vi "final16.vi"() -> ()   [LabVIEW 2019]
uses:
  <vilib>/Instr/_visa.llb/VISA Configure Serial Port (Instr).vi
  <vilib>/Analysis/NI_AALPro.lvlib
  <vilib>/Analysis/NI_AALBase.lvlib
panel:
  out "residue_gain0":dbl
  out "residue_gain2":dbl
  out "residue_gain1":dbl
  out "Received data":string
  out "initialized array":dbl[](array[numeric])
  out "standard deviation":dbl format="%0.2f"
  out "variance":dbl format="%0.2f"
  out "mean":dbl format="%0.2f"
  out "Conversion [g]":dbl
  out "slope_gain0":dbl
  out "intercept_gain0":dbl
  out "slope_gain2":dbl
  out "intercept_gain2":dbl
  out "slope_gain1":dbl
  out "intercept_gain1":dbl
  out "Debug array":string[](array[string])
  in  "Stop":bool
  in  "Cycles":dbl min=1.0 step=1.0
  in  "Start operation":bool
  out "String passed to Arduino":string
  in  "Function":u16(ring) items=["Read data ", "Compare different gains", "Execute calibration"]
  in  "Gain":u16(ring) items=["32", "64", "128"]
  in  "Arduino COM port":refnum<visa-resource-name>="COM6"
  # "Select all options, then press \"Start operation\" button"
  # "Nerd zone"
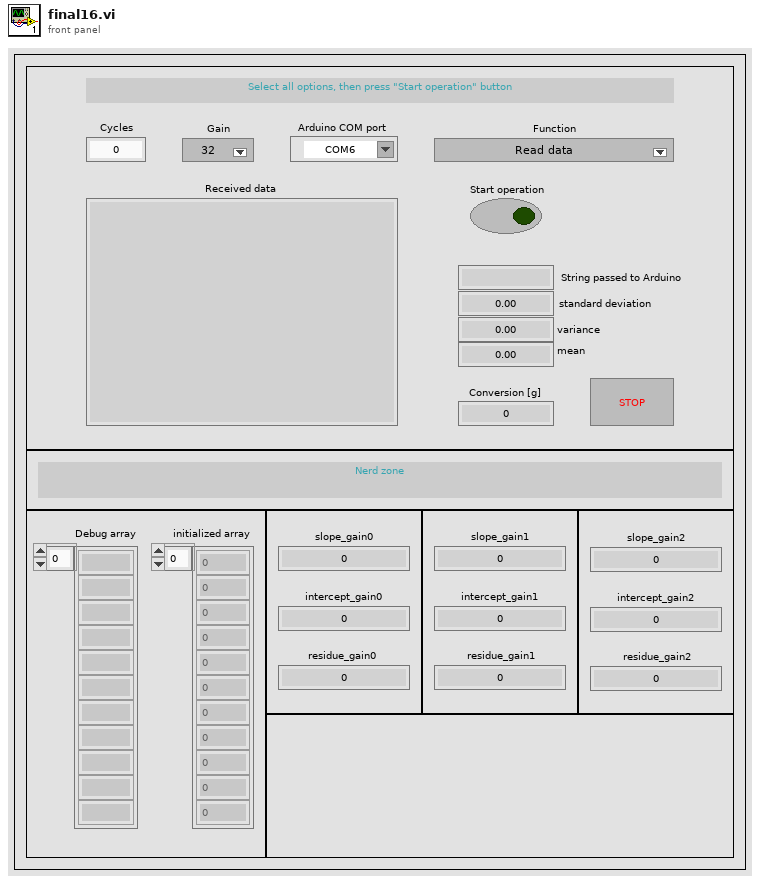
[diagram p1: front panel]
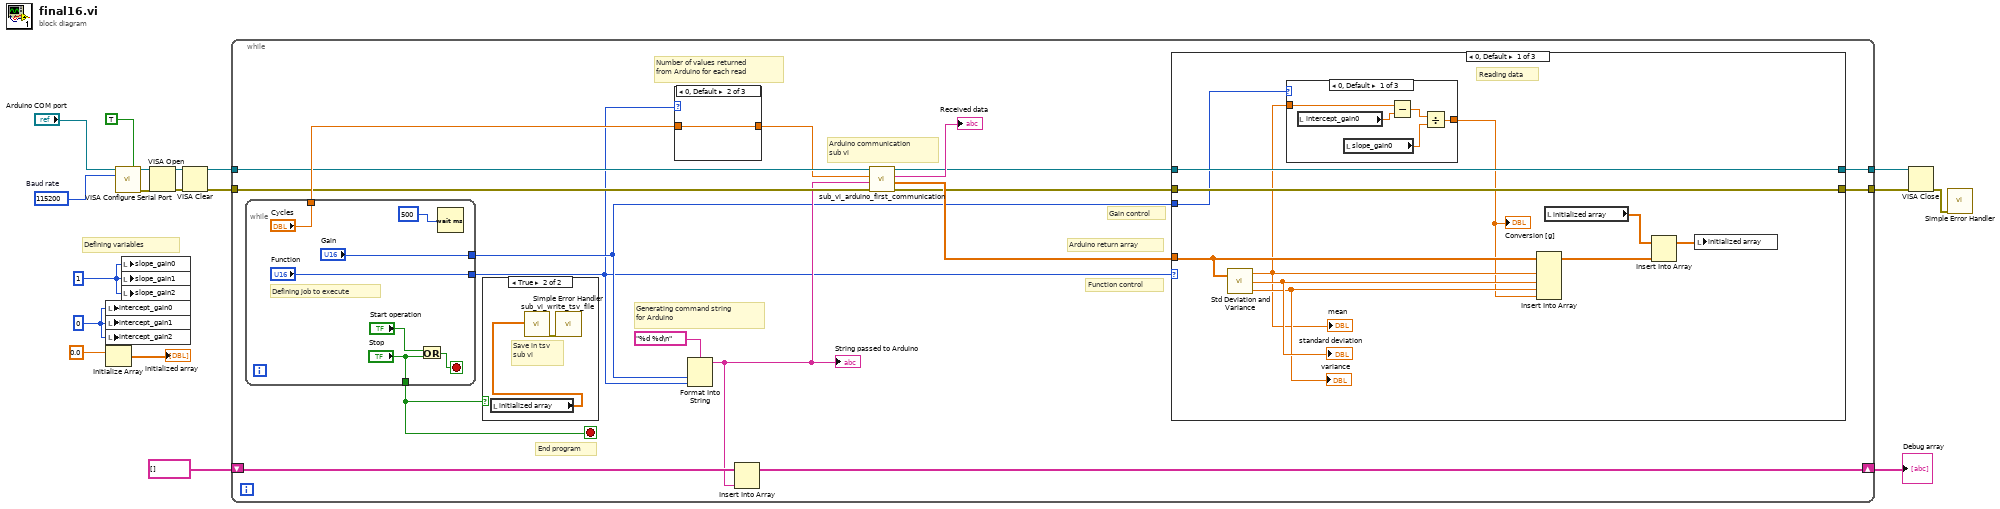
[diagram p0: block diagram]
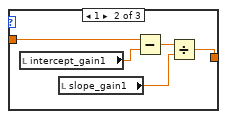
[diagram p2: hidden frame]
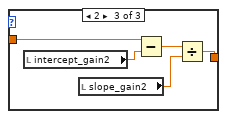
[diagram p3: hidden frame]
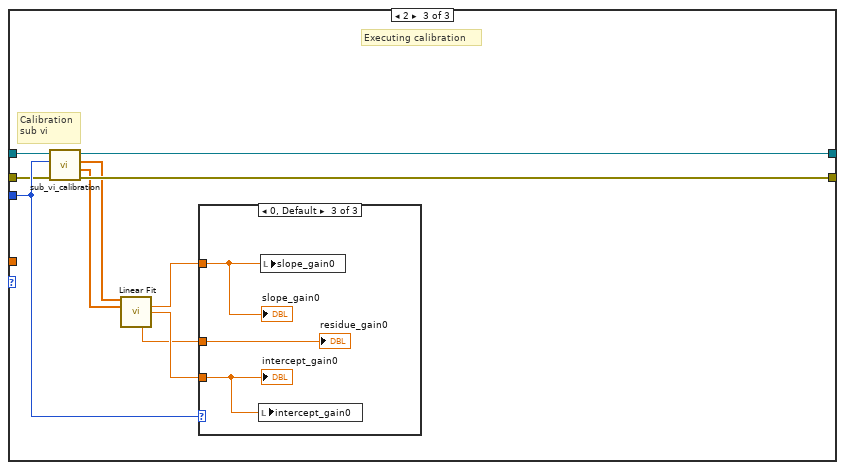
[diagram p5: hidden frame]
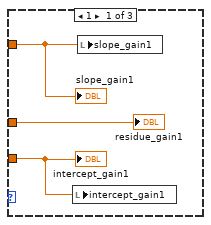
[diagram p6: hidden frame]
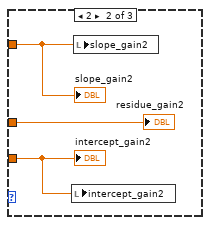
[diagram p7: hidden frame]
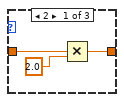
[diagram p8: hidden frame]
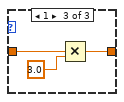
[diagram p9: hidden frame]
diagram:
  w6 = 0
  w5 = 1
  w17 = u32 115200  # Baud rate
  # "Defining variables"
  n1 = local write "intercept_gain0"(w6) -> ()
  n2 = local write "intercept_gain1"(w6) -> ()
  n3 = local write "intercept_gain2"(w6) -> ()
  n4 = Initialize Array(0.0) -> (→"initialized array":dbl[])  [unwired: 1 in]
  n5 = call-poly "VISA Configure Serial Port"("VISA resource name"="Arduino COM port", "Enable Termination\nChar (T)"=TRUE ("Enable Termination\nChar (T)"), "baud rate (9600)"=w17) -> ("VISA resource name out"=w15:refnum<visa-resource-name>, "error out"=w16:errorcluster)  [unwired: 11 in]
  n6 = local write "slope_gain0"(w5) -> ()
  n7 = local write "slope_gain1"(w5) -> ()
  n8 = local write "slope_gain2"(w5) -> ()
  n9 = VISA Open(error in (no error)=w16, VISA resource name=w15) -> (VISA resource name=w12:refnum<visa-resource-name>, error out=w13:errorcluster)  [unwired: 3 in]
  n10 = VISA Clear(VISA resource name=w12, error in (no error)=w13) -> (VISA resource name out=w10:refnum<visa-resource-name>, error out=w11:errorcluster)
  n11 = while {
    tunnel: w11 -> [w29]
    tunnel: w10 -> [w30]
    shift-right: [w35] -> w8
    shift-left: string[] [] -> [w33]
    tunnel: [w21] -> w2
    tunnel: [w22] -> w1
    stop <- w34 stop-if-true
    # "Number of values returned \nfrom Arduino for each read"
    # "End program"
    # "Generating command string\nfor Arduino"
    # "Function control"
    # "Arduino return array"
    # "Gain control"
    # "Arduino communication\nsub vi"
    n12 = while {
      tunnel: ["Function"] -> w19
      tunnel: ["Gain"] -> w20
      tunnel: ["Cycles"] -> w32
      tunnel: ["Stop"] -> w34
      stop <- w93 stop-if-true
      # "Defining job to execute"
      n13 = Or(x="Start operation", y="Stop") -> (x .or. y?=w93:bool)
      n14 = Wait (ms)(milliseconds to wait=u32 500) -> ()  [unwired: 1 out]
    }
    n15 = case shown="True" w34 {
      frame False {
      }
      frame True {
        # "Save in tsv\nsub vi"
        n16 = local read "initialized array"() -> (w90:dbl[])
        n17 = call "sub_vi_write_tsv_file.vi"("1D data"=w90) -> ("error out"=w91:errorcluster)  [unwired: 10 in]
        n18 = call <vilib>:"Simple Error Handler.vi"("error in (no error)"=w91) -> ()  [unwired: 4 in, 5 out]
      }
    }
    n19 = case shown="0, Default" w19 {
      tunnel: w32 -> [w85 w86 w87]
      tunnel: [w83 w86 w88] -> w27
      frame 2 {
        n20 = Multiply(x=w85, y=2.0) -> (x*y=w83:dbl)
      }
      frame 0, Default {
      }
      frame 1 {
        n21 = Multiply(x=w87, y=3.0) -> (x*y=w88:dbl)
      }
    }
    n22 = Format Into String(format string="%d %d\n", w20, w19) -> (resulting string=w28:string)  [unwired: 2 in, 1 out]
    "String passed to Arduino" <- w28
    n23 = Insert Into Array(array=w33, new element=w28) -> (w35:string[])  [unwired: 1 in]
    n24 = call "sub_vi_arduino_first_communication.vi"("error in (no error)"=w29, "write buffer"=w28, "Reads number"=w27, "VISA resource name in"=w30) -> ("error out"=w23:errorcluster, "Reads array"=w25:dbl[], "Received data"=→"Received data":string, "VISA resource name out"=w24:refnum<visa-resource-name>)  [unwired: 4 in]
    n25 = case shown="0, Default" w19 {
      tunnel: w20 -> [w37 _ w69]
      tunnel: w25 -> [w46 _ _]
      tunnel: w24 -> [w40 w63 w70]
      tunnel: w23 -> [w39 w62 w68]
      tunnel: [w40 w63 w64] -> w22
      tunnel: [w39 w62 w67] -> w21
      frame 0, Default {
        # "Reading data"
        n26 = call <vilib>:"Std Deviation and Variance.vi"("X"=w46) -> ("mean"=w38:dbl, "standard deviation"=w45:dbl, "variance"=w44:dbl)  [unwired: 1 in]
        "standard deviation" <- w45
        "variance" <- w44
        "mean" <- w38
        n27 = case shown="0, Default" w37 {
          tunnel: [w50 w55 w60] -> w36
          tunnel: w38 -> [w47 w52 w57]
          frame 0, Default {
            n28 = local read "intercept_gain0"() -> (w49:dbl)
            n29 = local read "slope_gain0"() -> (w48:dbl)
            n30 = Subtract(x=w47, y=w49) -> (x-y=w51:dbl)
            n31 = Divide(x=w51, y=w48) -> (x/y=w50:dbl)
          }
          frame 1 {
            n32 = local read "intercept_gain1"() -> (w54:dbl)
            n33 = local read "slope_gain1"() -> (w53:dbl)
            n34 = Subtract(x=w52, y=w54) -> (x-y=w56:dbl)
            n35 = Divide(x=w56, y=w53) -> (x/y=w55:dbl)
          }
          frame 2 {
            n36 = local read "intercept_gain2"() -> (w59:dbl)
            n37 = local read "slope_gain2"() -> (w58:dbl)
            n38 = Subtract(x=w57, y=w59) -> (x-y=w61:dbl)
            n39 = Divide(x=w61, y=w58) -> (x/y=w60:dbl)
          }
        }
        "Conversion [g]" <- w36
        n40 = Insert Into Array(array=w46, new element #1=w38, new element #2=w45, new element #3=w44, new element #4=w36) -> (w41:dbl[])  [unwired: 1 in]
        n41 = local read "initialized array"() -> (w42:dbl[])
        n42 = Insert Into Array(array=w42, new element=w41) -> (w43:dbl[])  [unwired: 1 in]
        n43 = local write "initialized array"(w43) -> ()
      }
      frame 1 {
        # "Comparing different gains"
      }
      frame 2 {
        # "Calibration\nsub vi"
        # "Executing calibration"
        n44 = call "sub_vi_calibration.vi"("error in (no error)"=w68, "Gain"=w69, "VISA resource name"=w70) -> ("error out"=w67:errorcluster, "Weights"=w66:dbl[], "Measures"=w65:dbl[], "VISA resource name out"=w64:refnum<visa-resource-name>)  [unwired: 5 in]
        n45 = call <vilib>:"Linear Fit.vi"("Y"=w65, "X"=w66) -> ("slope"=w73:dbl, "intercept"=w72:dbl, "residue"=w71:dbl)  [unwired: 9 in, 2 out]
        n46 = case shown="0, Default" w69 {
          tunnel: w73 -> [w76 w79 w82]
          tunnel: w72 -> [w75 w78 w81]
          tunnel: w71 -> [w74 w77 w80]
          frame 1 {
            n47 = local write "intercept_gain1"(w75) -> ()
            n48 = local write "slope_gain1"(w76) -> ()
            "slope_gain1" <- w76
            "intercept_gain1" <- w75
            "residue_gain1" <- w74
          }
          frame 2 {
            n49 = local write "intercept_gain2"(w78) -> ()
            n50 = local write "slope_gain2"(w79) -> ()
            "slope_gain2" <- w79
            "intercept_gain2" <- w78
            "residue_gain2" <- w77
          }
          frame 0, Default {
            n51 = local write "intercept_gain0"(w81) -> ()
            n52 = local write "slope_gain0"(w82) -> ()
            "slope_gain0" <- w82
            "intercept_gain0" <- w81
            "residue_gain0" <- w80
          }
        }
      }
    }
  }
  "Debug array" <- w8
  n53 = VISA Close(VISA resource name=w1, error in (no error)=w2) -> (error out=w7:errorcluster)
  n54 = call <vilib>:"Simple Error Handler.vi"("error in (no error)"=w7) -> ()  [unwired: 4 in, 5 out]
